vi "Regulation v2.vi"(6 "PID Cluster":T2={"L1 to L4 PID Cluster"={"L1 PID Gains"={"Kp"=0.005, "Kd"=0.5, "Ki"=0.0005}, "L2 PID Gains"={"Kp"=0.01, "Kd"=1.0, "Ki"=0.005}, "L3 PID Gains"={"Kp"=0.05, "Kd"=1.0, "Ki"=0.0005}, "L4 PID Gains"={"Kp"=0.1, "Kd"=0.1, "Ki"=0.0005}}, "Stage PID Cluster"={"Stage Z PID"={"Kp"=0.0005, "Kd"=0.001, "Ki"=0.0}, "Stage Y PID"={"Kp"=0.0003, "Kd"=0.01, "Ki"=0.0}, "Stage X PID"={"Kp"=0.0003, "Kd"=0.01, "Ki"=0.0}}, "OCT Z PID Gains"={"Kp"=0.0003, "Kd"=0.0001, "Ki"=0.01}}, 7 "Robot In":i32, 8 "error in":errorcluster, 9 "Engage Pt":dbl[](array[numeric])=[0.0, 0.0, 0.0, 0.0], 10 "Prev Posit Cluster":T3={"Prev L1 to L4 Posit"=[0.0, 0.0, 0.0, 0.0], "Prev Stage Posit"=[6.0, 6.0, 6.0], "Prev OCT Z Posit"=0.0}, 11 "FPGA VI Reference In":refnum<k20>) -> (0 "error out":errorcluster, 2 "Last Posit Cluster":T1={"Last L1 to L4 Posit"=[0.0, 0.0, 0.0, 0.0], "Last Stage Posit"=[6.0, 6.0, 6.0], "Last OCT Z Posit"=0.0}, 3 "FPGA VI Reference Out":refnum<k20>)   [LabVIEW 2016]
uses:
  Subsystems/Global Variables.vi
  <vilib>/rvi/interface/nirviReadWriteControl/nirviReadWriteControl.xnode
  <vilib>/platform/TimedLoop/XDataNode/XDataNode.xnode
  <vilib>/Platform/TimedLoop/XDataNode/timing_clust.ctl
  <vilib>/Platform/TimedLoop/XDataNode/XDNodeRunTimeDep.lvlib
  <vilib>/Platform/TimedLoop/XDataNode/wakeup.ctl
  <vilib>/Platform/TimedLoop/XDataNode/nitl_modes.ctl
  FPGA Bitfiles/PhantomControlPI_FPGATarget_QuadCtr2_E2412E44.lvbitx
  IRISS_FPGA_IO.vi
  NiFpgaLv.dll
  <vilib>/Utility/error.llb/Error Cluster From Error Code.vi
  <vilib>/rvi/errors/niLvFpgaAdjustHostInterfaceError.vi
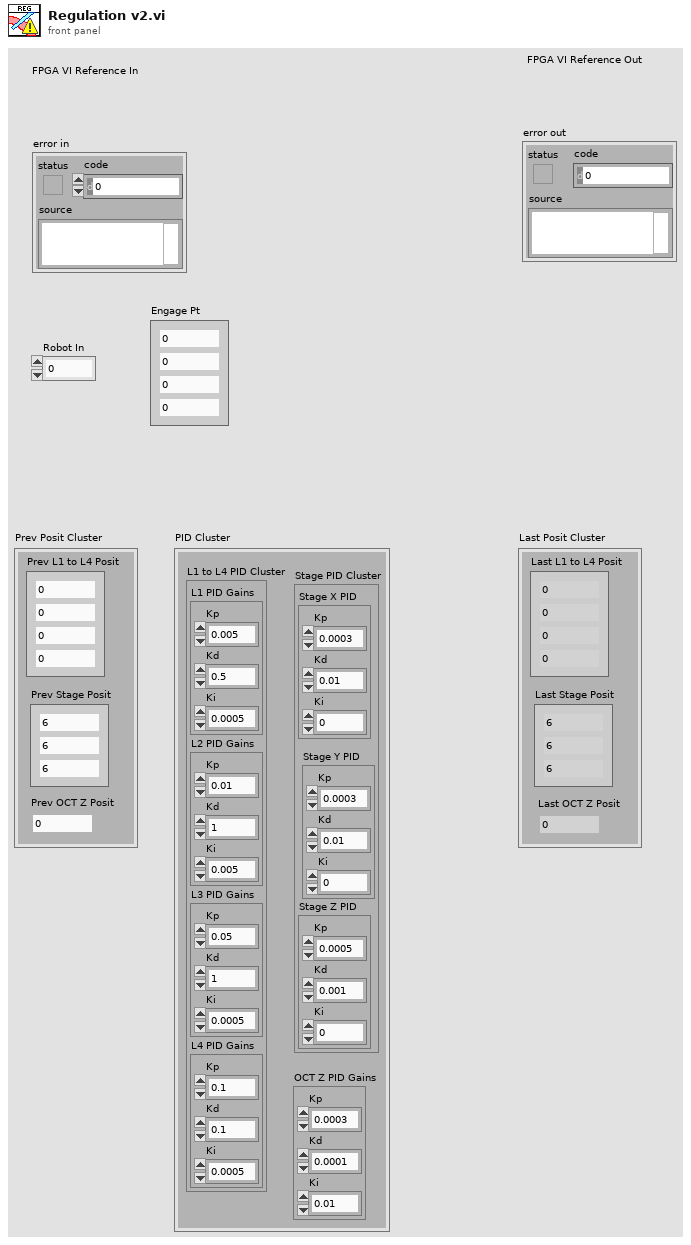
[diagram p1: front panel]
types:
  T1 = cluster{"Last L1 to L4 Posit":dbl[], "Last Stage Posit":dbl[], "Last OCT Z Posit":dbl}
  T2 = cluster{"L1 to L4 PID Cluster":cluster{"L1 PID Gains":cluster{"Kp":dbl, "Kd":dbl, "Ki":dbl}, "L2 PID Gains":cluster{"Kp":dbl, "Kd":dbl, "Ki":dbl}, "L3 PID Gains":cluster{"Kp":dbl, "Kd":dbl, "Ki":dbl}, "L4 PID Gains":cluster{"Kp":dbl, "Kd":dbl, "Ki":dbl}}, "Stage PID Cluster":cluster{"Stage Z PID":cluster{"Kp":dbl, "Kd":dbl, "Ki":dbl}, "Stage Y PID":cluster{"Kp":dbl, "Kd":dbl, "Ki":dbl}, "Stage X PID":cluster{"Kp":dbl, "Kd":dbl, "Ki":dbl}}, "OCT Z PID Gains":cluster{"Kp":dbl, "Kd":dbl, "Ki":dbl}}
  T3 = cluster{"Prev L1 to L4 Posit":dbl[], "Prev Stage Posit":dbl[], "Prev OCT Z Posit":dbl}
  T4 = typedef "XDNodeRunTimeDep.lvlib/timing_clust.ctl" = cluster{"Expected End [f-1]":u64, "Actual End [f-1]":u64, "Finished Late? [f-1]":bool, "Expected End [i-1]":u64, "Actual End [i-1]":u64, "Finished Late? [i-1]":bool, "Expected Start [i]":u64, "Actual Start [i]":u64, "Expected Start [f]":u64, "Actual Start [f]":u64, "Source Name":string, "Structure Name":string, "Period":i64, "Deadline":i64, "Offset":i64, "Start":i64, "Priority":i32, "Timeout":i32, "Mode":T5, "Wakeup Reason":T6, "Error":errorcluster, "Source Type":string, "Secondary Source Type":string, "Global End Time":u64, "Global Start Time":u64, "Frame Duration":u64, "Iteration Duration":u64, "Assigned CPU":i32, "I/O Scan Engine Mode":u32}
  T5 = typedef "XDNodeRunTimeDep.lvlib/nitl_modes.ctl" = enum32{"No Change", "Process missed periods, maintain original phase", "Discard missed periods, maintain original phase", "Process missed periods, ignore original phase", "Discard missed periods, ignore original phase"}
  T6 = typedef "XDNodeRunTimeDep.lvlib/wakeup.ctl" = enum32{"Normal", "Aborted", "Asynchronous wakeup", "Timing source error", "Timed loop error", "Timeout"}
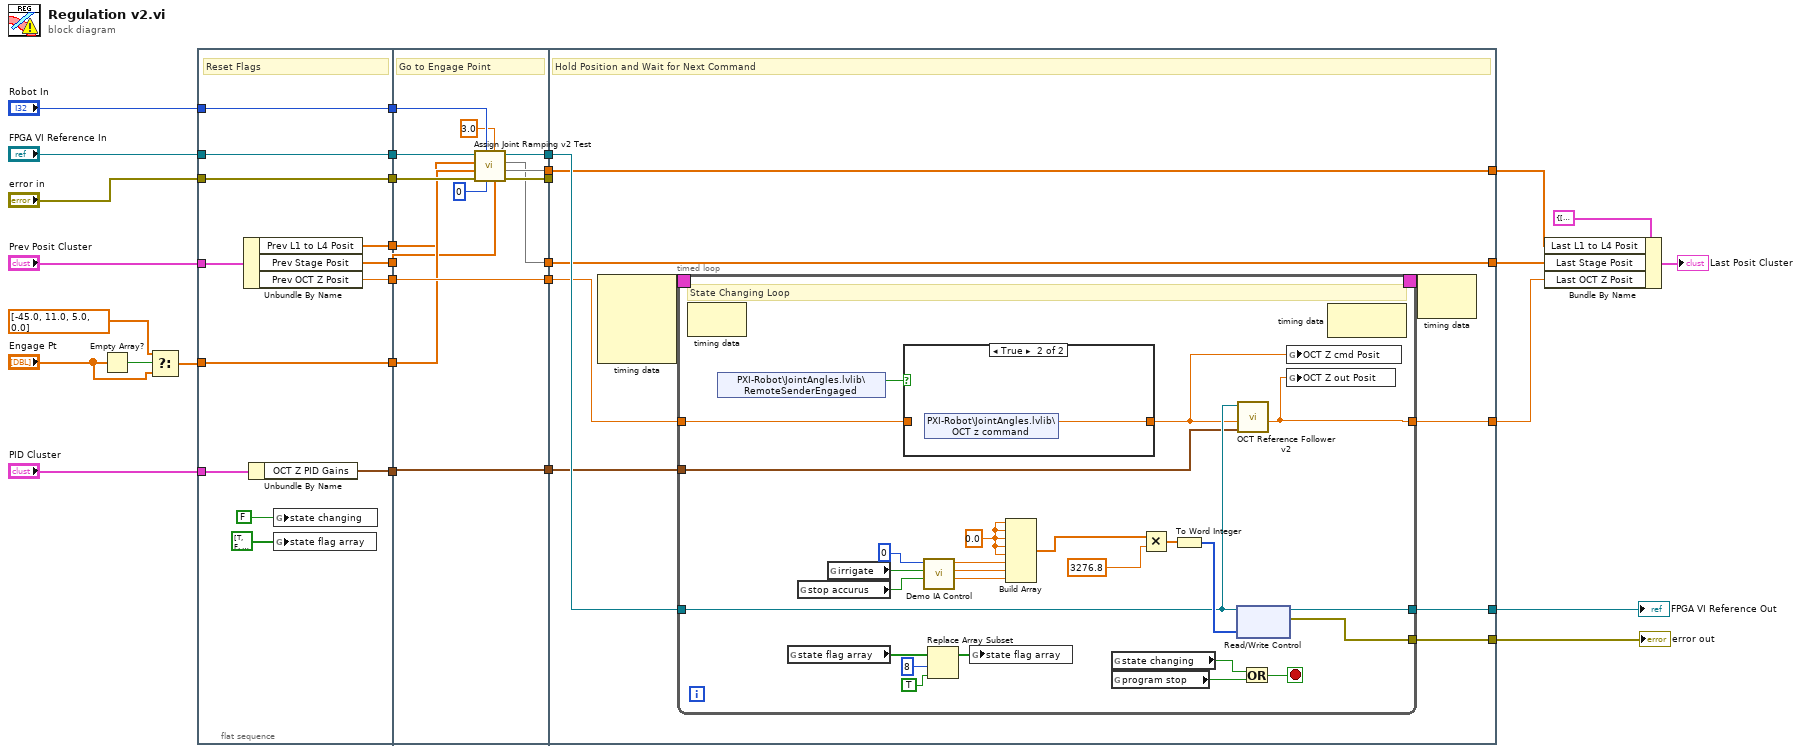
[diagram p0: block diagram]
diagram:
  n1 = Empty Array?(array="Engage Pt") -> (empty?=w24:bool)
  n2 = Select(t=dbl[] [-45.0, 11.0, 5.0, 0.0] ("First Trk Pt 2"), s=w24, f="Engage Pt") -> (s? t:f=w21:dbl[])
  n3 = flat-sequence {
    tunnel: [w40] -> w30
    tunnel: "FPGA VI Reference In" -> [w40]
    tunnel: "error in" -> [w39]
    tunnel: [w39] -> w29
    tunnel: [w35] -> w28
    tunnel: "PID Cluster" -> [w33]
    tunnel: [w34] -> w26
    tunnel: w21 -> [w34]
    tunnel: "Prev Posit Cluster" -> [w38]
    tunnel: [w37] -> w12
    tunnel: [w36] -> w9
    tunnel: [w32] -> w8
    tunnel: [w31] -> w6
    tunnel: "Robot In" -> [w31]
    tunnel: w30 -> [w55]
    tunnel: w29 -> [w52]
    tunnel: w28 -> [w50]
    tunnel: w26 -> [w51]
    tunnel: [w53] -> w25
    tunnel: [w54] -> w20
    tunnel: [w45] -> w18
    tunnel: w12 -> [w44]
    tunnel: [w43] -> w11
    tunnel: [w56] -> w10
    tunnel: w9 -> [w56]
    tunnel: w8 -> [w45]
    tunnel: w6 -> [w49]
    tunnel: [w47] -> w4
    tunnel: w25 -> [_]
    tunnel: w20 -> [w64]
    tunnel: [w60] -> w19
    tunnel: w18 -> [w58]
    tunnel: w11 -> [w60]
    tunnel: w10 -> [w63]
    tunnel: [w59] -> w7
    tunnel: w4 -> [w59]
    tunnel: [w62] -> w3
    tunnel: [w61] -> w2
    tunnel: [w57] -> w1
    frame #0 {
      # "Reset Flags"
      n4 = Unbundle By Name(w38) -> ("Prev L1 to L4 Posit"=w35:dbl[], "Prev Stage Posit"=w37:dbl[], "Prev OCT Z Posit"=w36:dbl)
      n5 = Unbundle By Name(w33) -> ("OCT Z PID Gains"=w32:cluster{"Kp":dbl, "Kd":dbl, "Ki":dbl})
      n6 = global write "Global Variables.vi" "state changing"(FALSE ("state changing")) -> ()
      n7 = global write "Global Variables.vi" "state flag array"(bool[] [TRUE, FALSE, FALSE, FALSE, FALSE, FALSE, FALSE, FALSE, FALSE] ("state flag array")) -> ()
    }
    frame #1 {
      # "Go to Engage Point"
      n8 = call "Assign Joint Ramping v2 Test.vi"(4:w44, "Ramp Time [sec]"=3.0, "Vac Digital Cmd"=i8 0, "Robot In"=w49, "error in"=w52, "Destination Posit Array [mm]"=w51, 10:w50, "FPGA VI Reference In"=w55) -> ("error out"=w53:errorcluster, 1:w47, 2:w43, "FPGA VI Reference Out"=w54:refnum<k20>)
    }
    frame #2 {
      # "Hold Position and Wait for Next Command"
      n9 = node-c288() -> (w66:T4)  [unwired: 4 in]
      n10 = timed-loop {
        timing: w66 -> [_]
        timing-out: [_] -> w65
        tunnel: w64 -> [w72]
        tunnel: w63 -> [w73]
        tunnel: [w70] -> w62
        tunnel: [w69] -> w61
        tunnel: w58 -> [w68]
        tunnel: [w67] -> w57
        stop <- w86 stop-if-true
        w81 = 0.0 ("element")
        # "State Changing Loop"
        n11 = node-c288() -> ()  [unwired: 1 in, 1 out]
        n12 = shared-variable "PXI-Robot\\JointAngles.lvlib\\RemoteSenderEngaged"() -> (w74:bool)  [unwired: 1 in, 1 out]
        n13 = global read "Global Variables.vi" "state flag array"() -> (w91:bool[])
        n14 = global read "Global Variables.vi" "stop accurus"() -> (w82:bool)
        n15 = global read "Global Variables.vi" "irrigate"() -> (w83:bool)
        n16 = case shown="True" w74 {
          tunnel: [w93 w94] -> w71
          tunnel: w73 -> [w93 _]
          frame False {
            # "Hold Position if not Engaged"
          }
          frame True {
            n17 = shared-variable "PXI-Robot\\JointAngles.lvlib\\OCT z command"() -> (w94:dbl)  [unwired: 1 in, 1 out]
          }
        }
        n18 = call "Demo IA Control.vi"("E-Stop Vacuum"=w82, "Irrigate?"=w83, "8bit integer"=i8 0) -> ("Accurus Engaged Vout"=w78:dbl, "Accurus ChB Vout"=w79:dbl, "Accurus ChA Vout"=w80:dbl)  [unwired: 6 in]
        n19 = Replace Array Subset(array=w91, new element=TRUE ("new element/subarray"), index=8) -> (w90:bool[])
        n20 = global write "Global Variables.vi" "state flag array"(w90) -> ()
        n21 = Build Array(w81, w81, w81, w81, w81, w80, w79, w78) -> (w77:dbl[])
        n22 = global read "Global Variables.vi" "state changing"() -> (w92:bool)
        n23 = global read "Global Variables.vi" "program stop"() -> (w87:bool)
        n24 = Multiply(x=w77, y=3276.8) -> (x*y=w85:dbl[])
        n25 = To Word Integer(number=w85) -> (16bit integer=w75:i16[])
        n26 = xnode "Read/Write Control"("FPGA VI Reference In"=w72, "AO"=w75) -> ("FPGA VI Reference Out"=w69:refnum<k20>, "error out"=w67:errorcluster)  [unwired: 1 in]
        n27 = call "OCT Reference Follower v2.vi"("OCT Z PID Gains"=w68, "OCT  Z cmd Posit [mm]"=w71, "FPGA VI Reference In"=w72) -> ("OCT  Z out Posit [mm]"=w70:dbl)  [unwired: 6 in, 2 out]
        n28 = Or(x=w92, y=w87) -> (x .or. y?=w86:bool)
        n29 = global write "Global Variables.vi" "OCT Z cmd Posit"(w71) -> ()
        n30 = global write "Global Variables.vi" "OCT Z out Posit"(w70) -> ()
        n31 = node-c288() -> ()  [unwired: 1 in, 1 out]
      }
      n32 = node-c288(w65) -> ()  [unwired: 1 out]
    }
  }
  n33 = Bundle By Name(cluster=T1 {"Last L1 to L4 Posit"=[0.0, 0.0, 0.0, 0.0], "Last Stage Posit"=[6.0, 6.0, 6.0], "Last OCT Z Posit"=0.0} ("Last Posit Cluster 2"), "Last L1 to L4 Posit"=w7, "Last Stage Posit"=w19, "Last OCT Z Posit"=w3) -> (→"Last Posit Cluster":T1)
  "FPGA VI Reference Out" <- w2
  "error out" <- w1
